vi "createInputStr.vi"(8 "error in (no error)":errorcluster, 9 "dataType":T1, 10 "data":variant, 11 "CoolerSerialCommand in":refnum<class "CoolerSerialCommand.lvclass">) -> (0 "error out":errorcluster, 2 "cmdDataStr":string, 3 "CoolerSerialCommand out":refnum<class "CoolerSerialCommand.lvclass">)   [LabVIEW 2016, in "CoolerSerialCommand.lvclass"]
uses:
  CoolerSerialCommand.lvclass
  dataType.ctl
  ControlSensor.ctl
  ExternalSensorStatus.ctl
  ChillerStatus.ctl
panel:
  out "length":i32
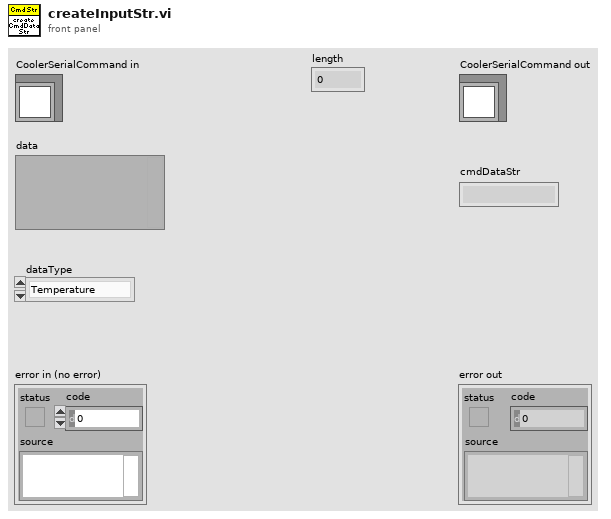
[diagram p1: front panel]
types:
  T1 = typedef "dataType.ctl" = enum16{"Temperature", "Flow", "ControlSensor", "ExternalSensorStatus", "ChillerStatus"}
  T2 = typedef "ControlSensor.ctl" = enum16{"SupplyTemperature", "ReturnTemperature", "ExtRTD", "ExternalTermistor"}
  T3 = typedef "ExternalSensorStatus.ctl" = enum16{"Disabled", "Enabled"}
  T4 = typedef "ChillerStatus.ctl" = enum16{"StandBy", "Run"}
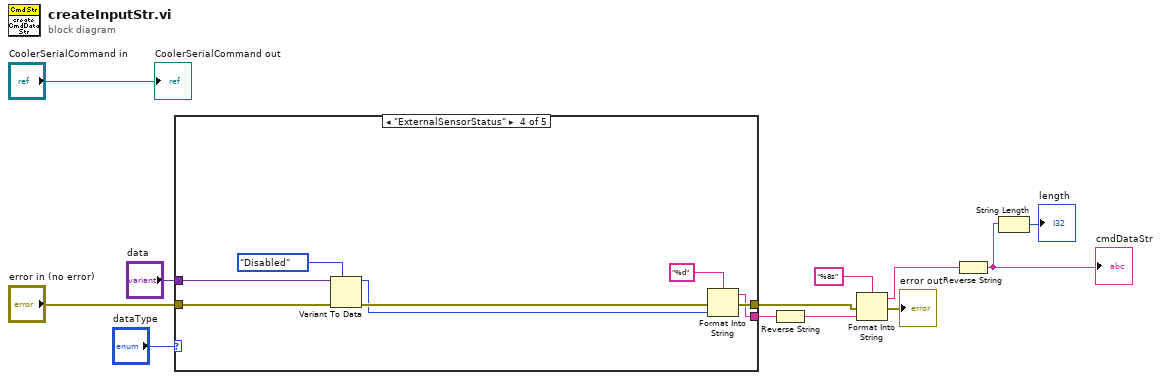
[diagram p0: block diagram]
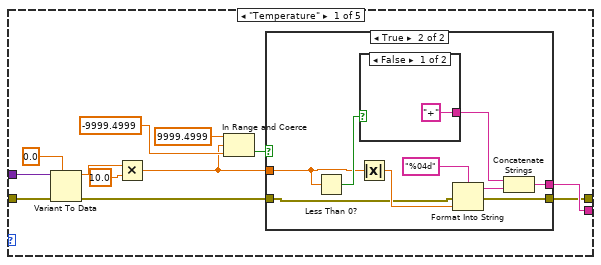
[diagram p2: hidden frame]
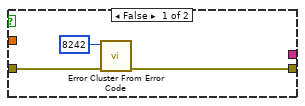
[diagram p3: hidden frame]
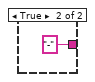
[diagram p4: hidden frame]
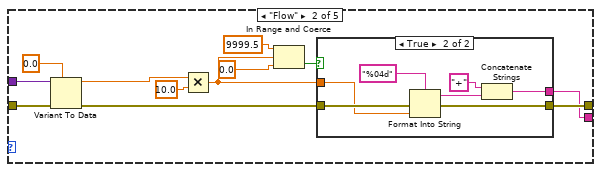
[diagram p5: hidden frame]
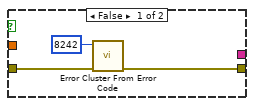
[diagram p6: hidden frame]
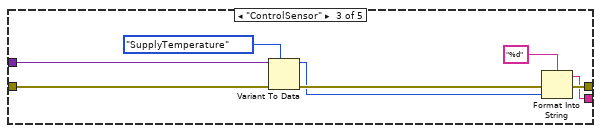
[diagram p7: hidden frame]
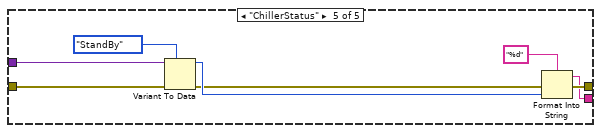
[diagram p8: hidden frame]
diagram:
  n1 = case shown="\"ExternalSensorStatus\"" "dataType" {
    tunnel: "data" -> [w23 w50 w68 w76 w84]
    tunnel: "error in (no error)" -> [w24 w49 w67 w75 w83]
    tunnel: [w20 w45 w61 w69 w77] -> w6
    tunnel: [w15 w46 w64 w70 w78] -> w1
    frame "Temperature" {
      n2 = Variant To Data(error in=w24, type=0.0, Variant=w23) -> (data=w14:dbl, error out=w17:errorcluster)
      n3 = Multiply(x=w14, y=10.0) -> (x*y=w13:dbl)
      n4 = In Range and Coerce(upper limit=9999.4999, x=w13, lower limit=-9999.4999) -> (In Range?=w16:bool)  [unwired: 1 out]
      n5 = case shown="True" w16 {
        tunnel: [_ w32] -> w20
        tunnel: w13 -> [_ w28]
        tunnel: w17 -> [w26 w30]
        tunnel: [w25 w29] -> w15
        frame False {
          n6 = call <vilib>:"Error Cluster From Error Code.vi"("error in (no error)"=w26, "error code (0)"=8242) -> ("error out"=w25:errorcluster)  [unwired: 7 in]
        }
        frame True {
          n7 = Less Than 0?(x=w28) -> (x < 0?=w34:bool)
          n8 = Absolute Value(x=w28) -> (abs(x)=w31:dbl)
          n9 = case shown="False" w34 {
            tunnel: ["+" ("string") "-" ("string")] -> w33
            frame False {
            }
            frame True {
            }
          }
          n10 = Format Into String(format string="%04d", error in=w30, w31) -> (resulting string=w35:string, error out=w29:errorcluster)  [unwired: 1 in]
          n11 = Concatenate Strings(w33, w35) -> (w32:string)
        }
      }
    }
    frame "Flow" {
      n12 = Variant To Data(error in=w49, type=0.0, Variant=w50) -> (data=w43:dbl, error out=w47:errorcluster)
      n13 = Multiply(x=w43, y=10.0) -> (x*y=w42:dbl)
      n14 = In Range and Coerce(upper limit=9999.5, x=w42, lower limit=0.0) -> (In Range?=w39:bool)  [unwired: 1 out]
      n15 = case shown="True" w39 {
        tunnel: w47 -> [w53 w59]
        tunnel: [w52 w58] -> w46
        tunnel: [_ w56] -> w45
        tunnel: w42 -> [_ w54]
        frame False {
          n16 = call <vilib>:"Error Cluster From Error Code.vi"("error in (no error)"=w53, "error code (0)"=8242) -> ("error out"=w52:errorcluster)  [unwired: 7 in]
        }
        frame True {
          n17 = Format Into String(format string="%04d", error in=w59, w54) -> (resulting string=w57:string, error out=w58:errorcluster)  [unwired: 1 in]
          n18 = Concatenate Strings("+" ("string"), w57) -> (w56:string)
        }
      }
    }
    frame "ControlSensor" {
      n19 = Variant To Data(error in=w67, type=ControlSensor."SupplyTemperature" ("ControlSensor"), Variant=w68) -> (data=w63:T2, error out=w65:errorcluster)
      n20 = Format Into String(format string="%d", error in=w65, w63) -> (resulting string=w61:string, error out=w64:errorcluster)  [unwired: 1 in]
    }
    frame "ExternalSensorStatus" {
      n21 = Variant To Data(error in=w75, type=ExternalSensorStatus."Disabled" ("ExternalSensorStatus"), Variant=w76) -> (data=w71:T3, error out=w72:errorcluster)
      n22 = Format Into String(format string="%d", error in=w72, w71) -> (resulting string=w69:string, error out=w70:errorcluster)  [unwired: 1 in]
    }
    frame "ChillerStatus" {
      n23 = Variant To Data(error in=w83, type=ChillerStatus."StandBy" ("ChillerStatus"), Variant=w84) -> (data=w80:T4, error out=w79:errorcluster)
      n24 = Format Into String(format string="%d", error in=w79, w80) -> (resulting string=w77:string, error out=w78:errorcluster)  [unwired: 1 in]
    }
  }
  n25 = Reverse String(1:w6) -> (0:w5:string)
  n26 = Format Into String(format string="%8s", error in=w1, w5) -> (resulting string=w4:string, error out=→"error out":errorcluster)  [unwired: 1 in]
  n27 = Reverse String(1:w4) -> (0:w3:string)
  "cmdDataStr" <- w3
  n28 = String Length(string=w3) -> (length=→"length":i32)
  "CoolerSerialCommand out" <- "CoolerSerialCommand in"
